vi "DebugProg.vi"() -> ()   [LabVIEW 2010]
uses:
  Instance           5 17Saved   DebugProg .vi
panel:
  out "Array":u8[](array[numeric])
  out "Result Input FOR VOC":u8[](array[numeric])
  out "ALG MSG  PARAM 2":enum16{"void", "byte", "int", "float"}(ring)
  out "Output varables names":string[](array[string])
  out "Output varables type":string[](array[string])
  out "AY Input varables names":string[](array[string])
  out "AY Input varables type":string[](array[string])
  out "Output ALG Msg Last Iter":string[][](table)=[["CODE", "PARAM"]]
  out "Output VOC Msg Last Iter":string[][](table)=[["CODE", "PARAM"]]
  out "Curr step ALG msg counter":i32
  out "Curr step VOC MSG counter":i32
  in  "Mode":bool
  in  "stop 2":bool
  in  "run":bool
  in  "Tab Control":T1(tab)=enum."Output ALG Info"
  out "ALG MSG queue":i32(slide) scale=0.0..5.0
  in  "send ALG msg":bool
  in  "ALG MSG  PARAM":string
  in  "ALG MSG  CODE":string(combo)="1"
  out "VOC MSG queue":i32(slide) scale=0.0..5.0
  in  "send voc msg 2":bool
  in  "VOC MSG  PARAM":string
  in  "VOC MSG  CODE":string(combo)
  in  "ALG MSG  TYPE":enum16{"void", "byte", "int", "float"}(ring)
  in  "VOC MSG  TYPE":enum16{"void", "byte", "int", "float"}(ring)
  out "AY OUTPUT Variables":string[][](table)
  in  "AY INPUT Variables":string[][](table)
  in  "New value\n(ALG ports)":u8
  in  "Controlable\n(ALG ports)":bool
  in  "Set new value\n(ALG ports)":bool
  in  "ALG Input Ports":i32(listbox)
  out "VOC OUTPUT Variables":string[][](table)
  in  "New value (VOC ports)":u8
  in  "Controlable (VOC ports)":bool
  in  "Set new value (VOC ports)":bool
  in  "VOC Input Ports":i32(listbox)
  in  "VOC INPUT Variables":string[][](table)
  in  "ALG Last Interation MSG":i32(listbox)
  out "Alg States":string[][](table)=[["Инициализация", "Начало", "0"], ["ОстановВсехПроцессовИстартПроцИнициализация", "Начало", "0"], ["КонтрольДостоверностиДавленияВбакеКомпрессора", "Начало", "0"], ["КонтрольДостоверностиДавленияВпатрубке", "Начало", "0"], ["КонтрольДостоверностиТемпературыВрубашкеОхлаждения", "Начало", "0"], ["КонтрольДостоверностиТемпературыВбакеОхлаждения", "Начало", "0"], ["КонтрольДостоверностиДавленияВтрубеСидеростата", "Начало", "0"], ["КонтрольДостоверностиСостоянияПитанияШКАФА_ВС", "Начало", "0"], ["КонтрольДостоверностиОткрЗатВакуумного", "Начало", "0"], ["КонтрольДостоверностиЗакрЗатВакуумного", "Начало", "0"], ["КонтрольДостоверностиСостоянияСапуна", "Начало", "0"], ["КонтрольДостоверностиСостоянияУстройстваПлавПуска", "Начало", "0"], ["КонтрольДостоверностиСостПитанияУППВакНасоса", "Начало", "0"], ["КонтрольДостоверностиСостоянияПитанияВентилятора", "Начало", "0"], ["КонтрольДостоверностиСостоянияПитанияРегТемпературы", "Начало", "0"], ["КонтрольДостоверностиСостоянияПитанияРегУровня", "Начало", "0"], ["КонтрольДостоверностиУровняВодыМинимум", "Начало", "0"], ["КонтрольДостоверностиУровняВодыМаксимум", "Начало", "0"], ["КонтрольДостоверностиСостоянияПитанияНасОхлаждения", "Начало", "0"], ["ЧтениеДавленияВбакеКомпрессора", "Начало", "0"], ["ОтлючитьВакуумированиеВручную", "ПереходВручноеОтключение", "0"], ["ЧтениеДавленияВпатрубке", "Начало", "0"], ["ЧтениеТемпературыВрубашкеОхлаждения", "Начало", "0"], ["ЧтениеТемпературыВбакеОхлаждения", "Начало", "0"], ["ЧтениеДавленияВтрубеСидеростата", "Начало", "0"], ["ПроверкаСвязиС_РегуляторомУровня", "Начало", "0"], ["ПроверкаСвязиС_РегуляторомТемпературы", "Начало", "0"], ["ПроверкаСвязиС_Вентилятором", "Начало", "0"], ["ПроверкаСвязиС_НасососомОхлажденияДвигателя", "Начало", "0"], ["ПроверкаСвязиС_КонцевикомОткрытияЗатвораВакуумного", "Начало", "0"], ["ПроверкаСвязиС_КонцевикомЗакрытияЗатвораВакуумного", "Начало", "0"], ["ПроверкаСвязиС_КонцевикомСапуна", "Начало", "0"], ["ПроверкаСвязиС_ПитаниемПлавногоПуска", "Начало", "0"], ["ПроверкаСвязиС_ПлавнымПуском", "Начало", "0"], ["РЕГУЛЯТОР_ТРАФИКА", "Начало", "0"], ["ЧтениеКольцевогоБуфера", "Начало", "0"], ["ОбработкаКомандИзмененияНП_от_ГУИ", "Анализ", "0"], ["ОбработкаКомандУправления_от_ГУИ", "Анализ", "0"], ["КонтрольИзменения_ФП_P_ВбакеКомпрессора", "Начало", "0"], ["КонтрольИзменения_ФП_P_Впатрубке", "Начало", "0"], ["КонтрольИзменения_ФП_T_Врубашке", "Начало", "0"], ["КонтрольИзменения_ФП_T_Вбаке", "Начало", "0"], ["КонтрольИзменения_ФП_P_ВтрубеСидер", "Начало", "0"], ["КонтрольВеличиныОткачкиВауумнойТрубыСидеростата", "Начало", "0"], ["КонтрольГотовностиВакуума_в_Вакуумной_Трубе", "Начало", "0"], ["КонтрольУровняВодыБакаОхлаждения", "Начало", "0"], ["КонтрольТемпературыВодыБакаОхлаждения", "Начало", "0"], ["КонтрольТемпературыРубашкиОхлаждения", "Начало", "0"], ["КонтрольДавленияВбакеКомпрессора", "Начало", "0"], ["КонтрольАварийногоДавленияВбакеКомпрессора", "Начало", "0"], ["КонтрольАварийнойТемпературыВрубашкеОхлаждения", "Начало", "0"], ["КонтрольАварийнойТемпературыВбакеОхлаждения", "Начало", "0"], ["КонтрольСостоянияПитанияШКАФА_ВС", "Начало", "0"], ["КонтрольСостоянияОборудования", "КонтрольОборудования", "0"], ["ВКЛ_ПИТ_ВЕНТИЛЯТОР", "Начало", "0"], ["ВЫК_ПИТ_ВЕНТИЛЯТОР", "Начало", "0"], ["КонтрольСостоянияПитанияВентилятора", "Начало", "0"], ["КонтрольСпонтанногоВыключенияВентилятора", "Контроль", "0"], ["КонтрольСпонтанногоВключенияВентилятора", "Контроль", "0"], ["КонтрольСостоянияЗатвораВакуумного", "Начало", "0"], ["ОТКР_ЗАТВОР_ВАК", "Начало", "0"], ["ЗАКР_ЗАТВОР_ВАК", "Начало", "0"], ["КонтрольСпонтанногоЗакрытияЗатвораВакуумного", "КонтрольЗакрытия", "0"], ["КонтрольСпонтанногоОткрытияЗатвораВакуумного", "Контроль", "0"], ["ОТКР_САПУН", "Начало", "0"], ["ЗАКР_САПУН", "Начало", "0"], ["КонтрольСостоянияПитанияСапуна", "Начало", "0"], ["КонтрольСпонтанногоЗакрытияСапуна", "КонтрольЗакрытия", "0"], ["КонтрольСпонтанногоОткрытияСапуна", "Контроль", "0"], ["ВКЛ_ПИТ_УПП_ВАК_НАСОСА", "Начало", "0"], ["ВЫК_ПИТ_УПП_ВАК_НАСОСА", "Начало", "0"], ["КонтрольСостоянияПитанияУППВакНасоса", "Начало", "0"], ["КонтрольСпонтанногоВыключенияУППВакНасоса", "Контроль", "0"], ["КонтрольСпонтанногоВключенияУППВакНасоса", "Контроль", "0"], ["ВКЛ_ПИТ_РЕГ_Т", "Начало", "0"], ["ВЫК_ПИТ_РЕГ_Т", "Начало", "0"], ["КонтрольСостоянияПитанияРЕГ_Т", "Начало", "0"], ["КонтрольСпонтанногоВыключенияРЕГ_Т", "Контроль", "0"], ["КонтрольСпонтанногоВключенияРЕГ_Т", "Контроль", "0"], ["ВКЛ_ПИТ_РЕГ_УР", "Начало", "0"], ["ВЫК_ПИТ_РЕГ_УР", "Начало", "0"], ["КонтрольСостоянияПитанияРЕГ_УР", "Начало", "0"], ["КонтрольСпонтанногоВыключенияРЕГ_УР", "Контроль", "0"], ["КонтрольСпонтанногоВключенияРЕГ_УР", "Контроль", "0"], ["ВКЛ_ПИТ_НАС_ОХЛ", "Начало", "0"], ["ВЫК_ПИТ_НАС_ОХЛ", "Начало", "0"], ["КонтрольСостоянияПитанияНАС_ОХЛ", "Начало", "0"], ["КонтрольСпонтанногоВыключенияНасосаОхлаждения", "Контроль", "0"], ["КонтрольСпонтанногоВключенияНасосаОхлаждения", "Контроль", "0"], ["ВКЛ_УСТР_ПЛАВ_ПУСКА", "Начало", "0"], ["ВЫК_УСТР_ПЛАВ_ПУСКА", "Начало", "0"], ["КонтрольСостоянияПитанияПЛАВ_ПУСКА", "Начало", "0"], ["КонтрольСпонтанногоВыключенияПлавнПуска", "Контроль", "0"], ["КонтрольСпонтанногоВключенияПлавнПуска", "Контроль", "0"], ["ВКЛ_ВАКУУМИРОВАНИЕ_ТРУБЫ", "Начало", "0"], ["ВЫК_ВАКУУМИРОВАНИЕ_ТРУБЫ", "Начало", "0"], ["ВКЛ_ВАКУУМНЫЙ_НАСОС", "Начало", "0"], ["ВЫК_ВАКУУМНЫЙ_НАСОС", "Начало", "0"]]
  out "Output Alg Msg LOG":string[][](table)=[["CODE", "PARAM"]]
  in  "VOC Last Interation MSG":i32(listbox)
  out "Output VOC Msg LOG":string[][](table)=[["CODE", "PARAM"]]
  out "VOC States":string[][](table)
  in  "Save as new test":bool
  in  "Save changes in current test":bool
  in  "TEST":string="script_port: 8 /*index*/, 0 /* СЦЕНАРИЙ_ЛОГ_ВХОД_ПИТ_ВЕНТИЛЯТОРА*/ \r\nscript_port: 9 /*index*/, 0 /* СЦЕНАРИЙ_ЛОГ_ВХОД_ПИТ_РЕГ_Т*/ \r\nscript_port: 10 /*index*/, 0 /* СЦЕНАРИЙ_ЛОГ_ВХОД_НАС_ОХЛ*/ \r\nscript_port: 11 /*index*/, 0 /* СЦЕНАРИЙ_ЛОГ_ВХОД_ВАК_НАСОСА*/ \r\nscript_port: 12 /*index*/, 0 /* СЦЕНАРИЙ_ЛОГ_ВХОД_ЗАТВОР_ВАК*/ \r\nscript_port: 13 /*index*/, 0 /* СЦЕНАРИЙ_ЛОГ_ВХОД_САПУН*/ \r\nscript_port: 14 /*index*/, 0 /* СЦЕНАРИЙ_ЛОГ_ВХОД_УСТР_ПЛАВ_ПУСКА*/ \r\nscript_port: 15 /*index*/, 0 /* СЦЕНАРИЙ_ЛОГ_ВХОД_РЕГ_УР*/ \r\nscript_port: 16 /*index*/, 0 /* СЦЕНАРИЙ_ЛОГ_ВХОД_КОМПРЕССОР*/ \r\n\n\n\n\n\n\n\n"
  in  "Tests List":i32(listbox)
  in  "stop":bool
  # "STEP MODE"
  # "CONTINUOUS MODE"
  # "ALG MSG Generation"
  # "VOC MSG Generation"
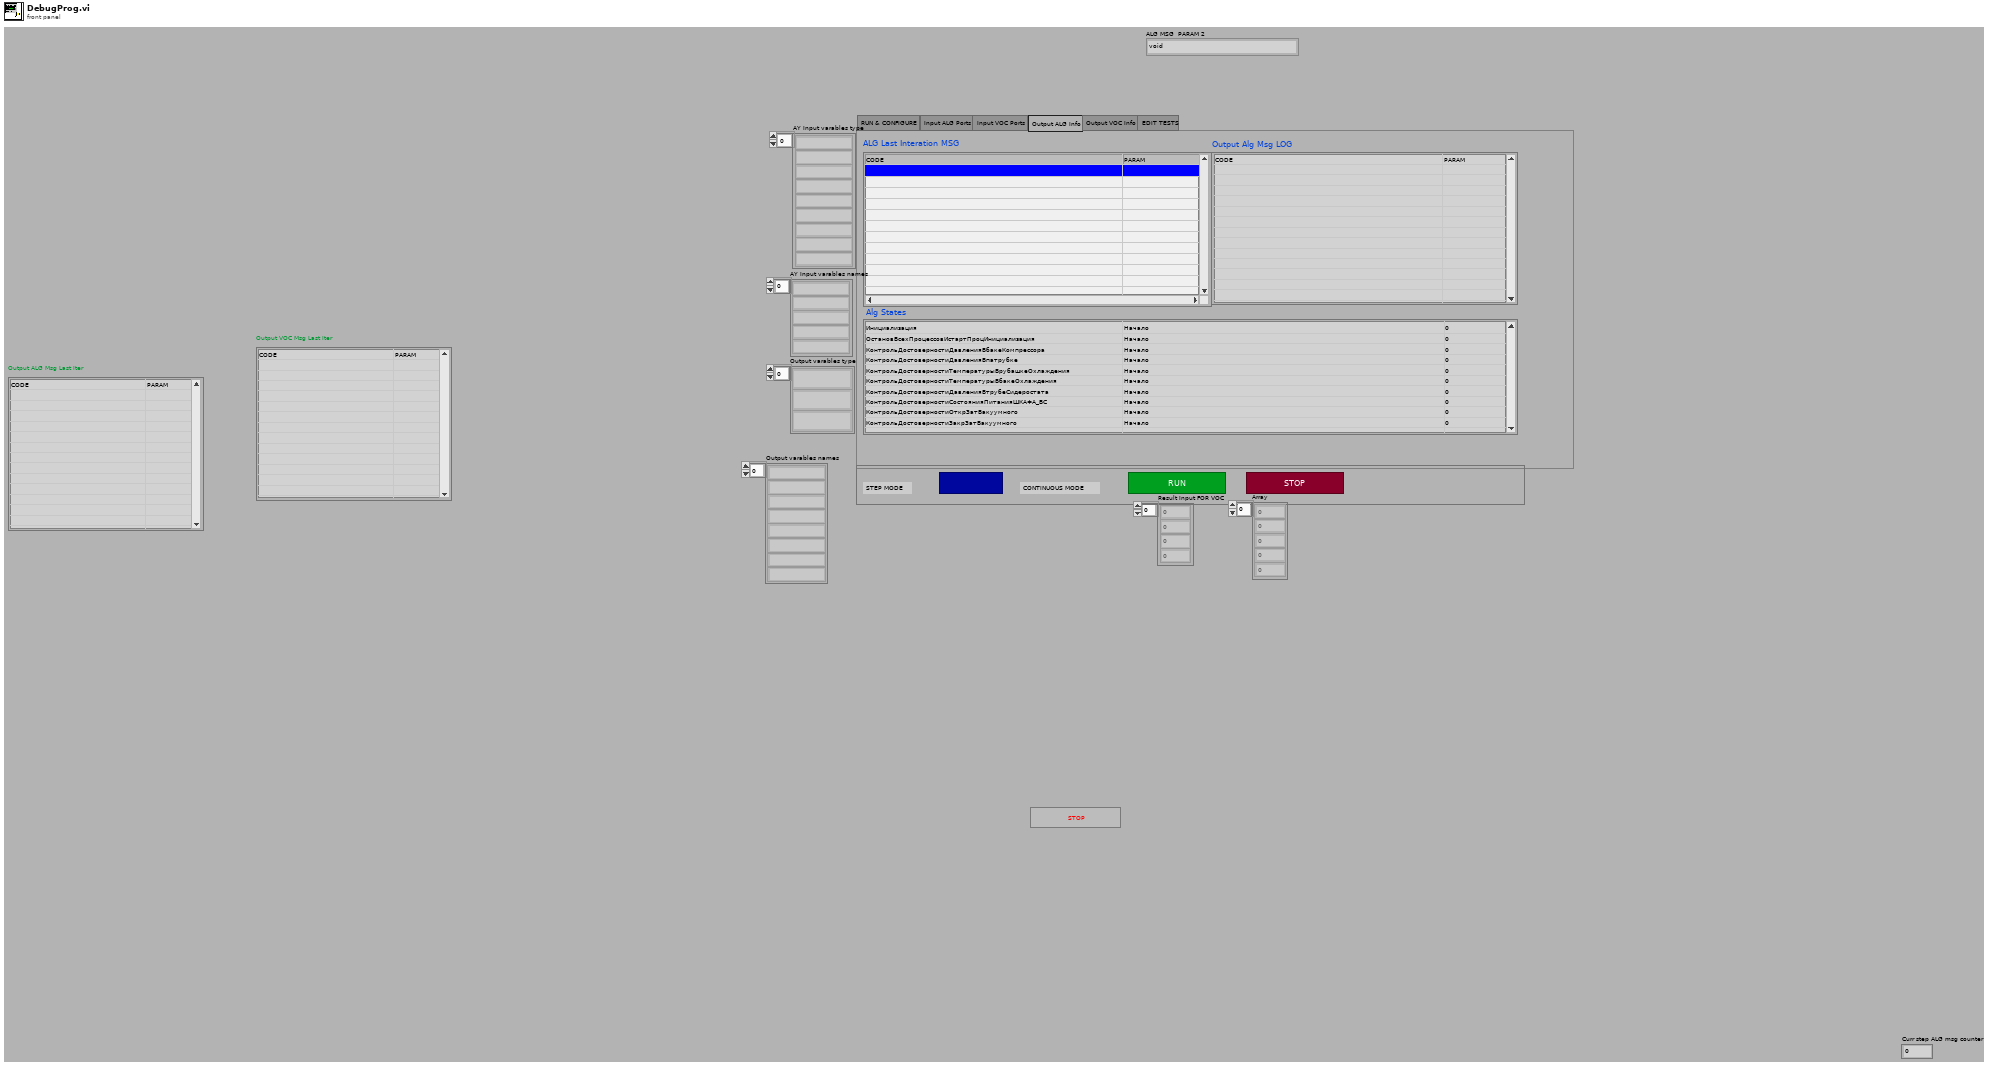
[diagram p1: front panel]
types:
  T1 = enum32{"RUN & CONFIGURE", "Input ALG Ports", "Input VOC Ports ", "Output ALG Info", "Output VOC Info", "EDIT TESTS"}
  T2 = enum8{"Enabled", "Disabled", "Disabled and Grayed Out"}
  T3 = enum16{"open", "open or create", "create or replace", "create", "open (read only)"}
  T4 = cluster{"code":i32, "param":i32, "Enum":enum16{"void", "byte", "int", "float"}}
  T5 = cluster{"trimmed string":string, "trimmed string":string}[]
  T6 = cluster{"code":i32, "param":i32, "Enum":enum16{"void", "byte", "int", "float"}}[]
  T7 = cluster{i32, "Casted Parameter":i32, "ALG MSG  TYPE":enum16{"void", "byte", "int", "float"}}
  T8 = cluster{i32, "Casted Parameter":i32, "VOC MSG  TYPE":enum16{"void", "byte", "int", "float"}}
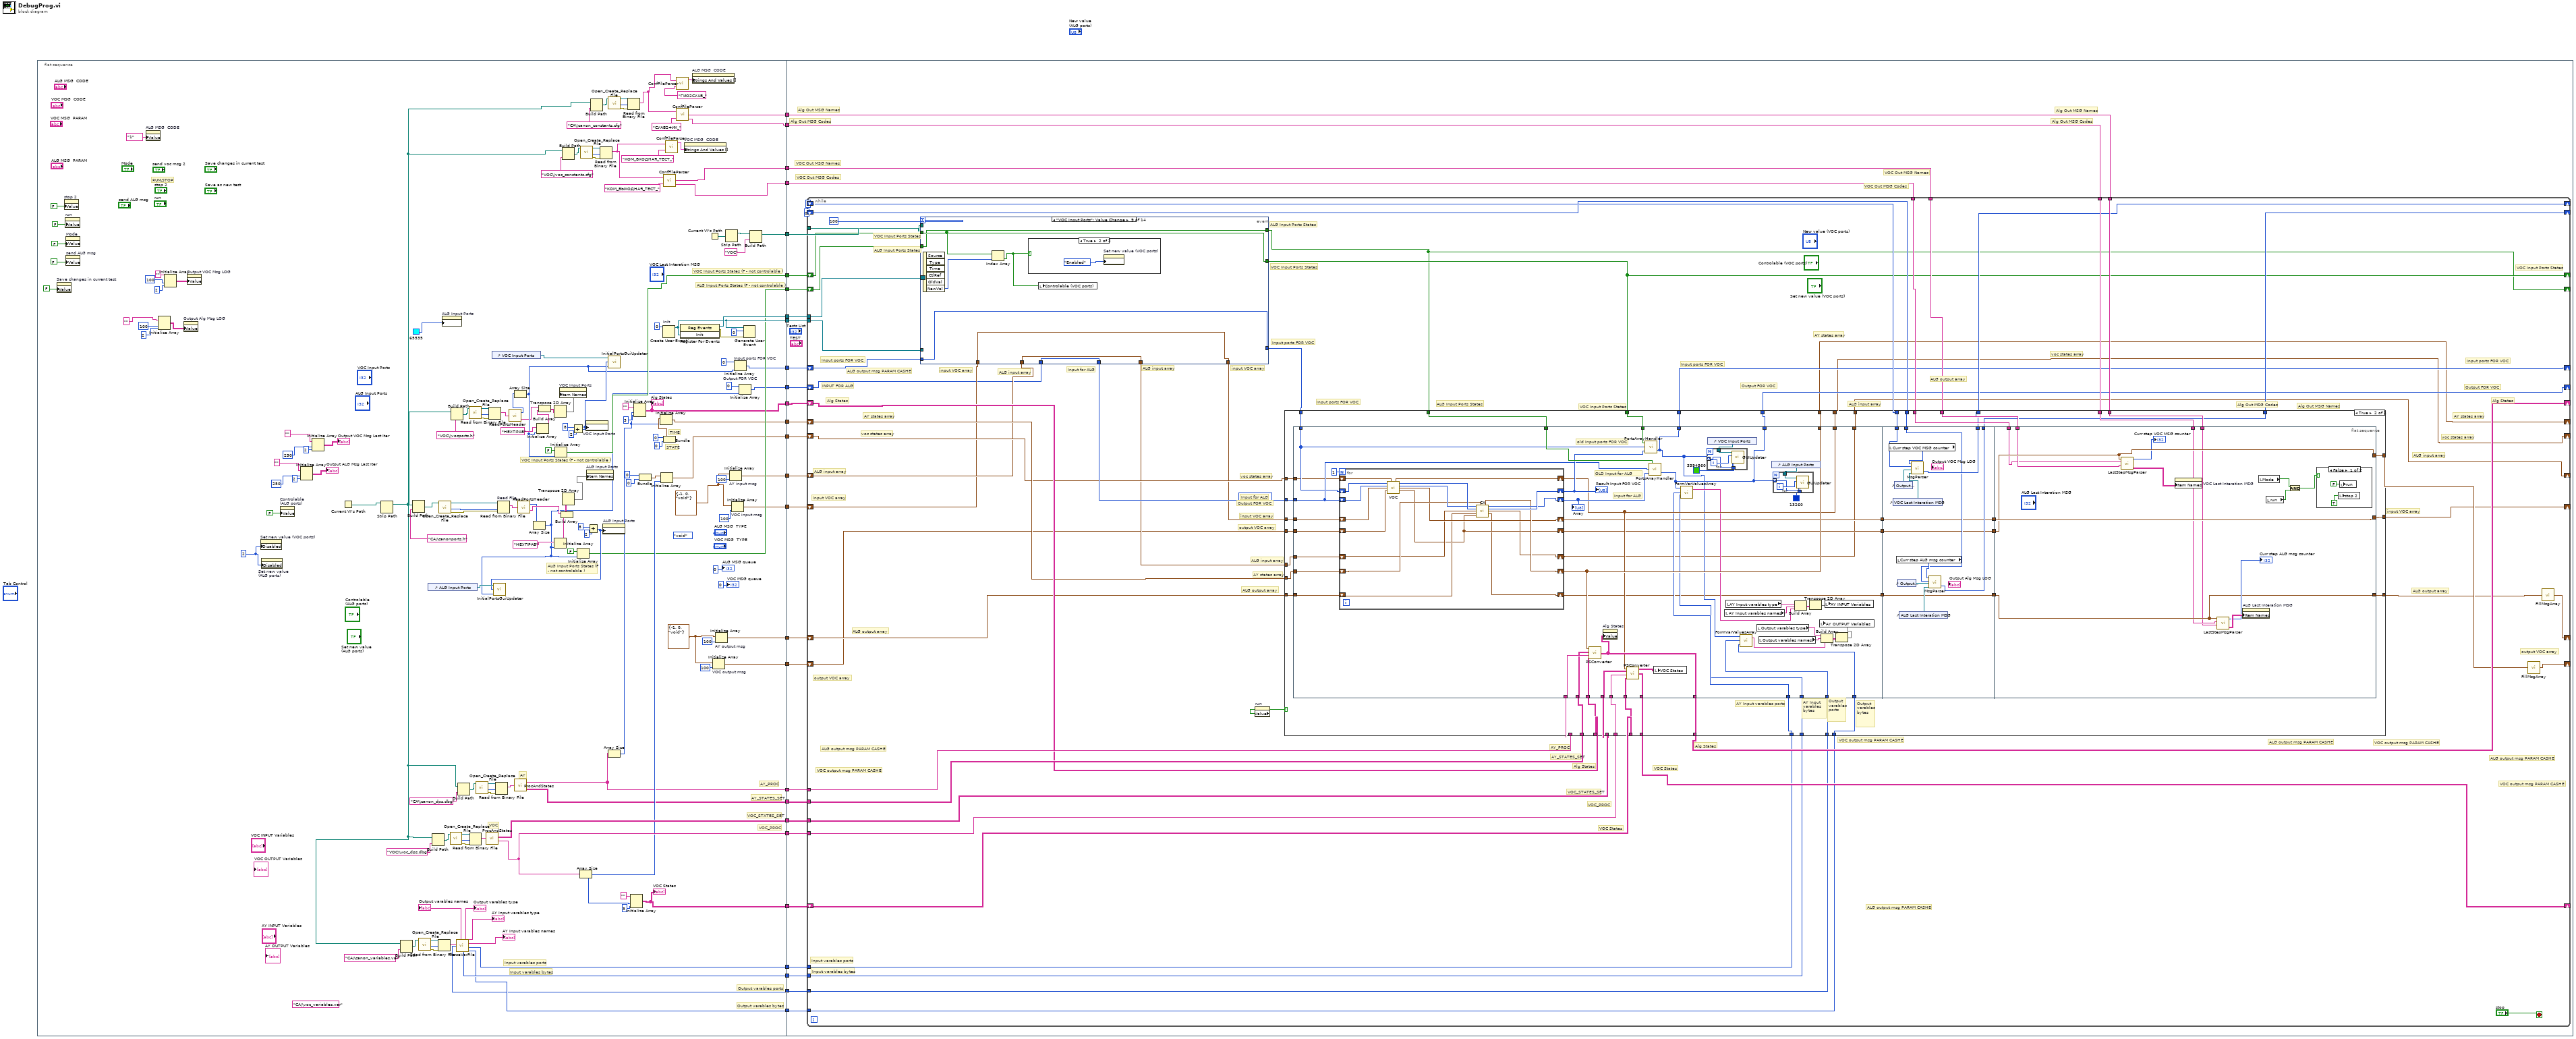
[diagram p0: block diagram]
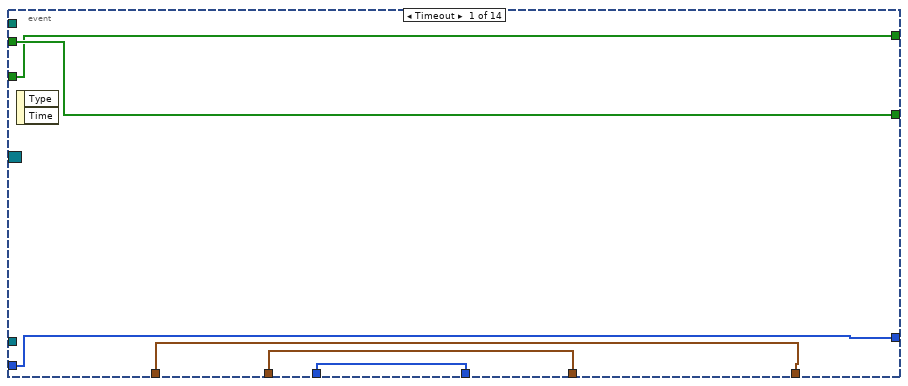
[diagram p2: hidden frame]
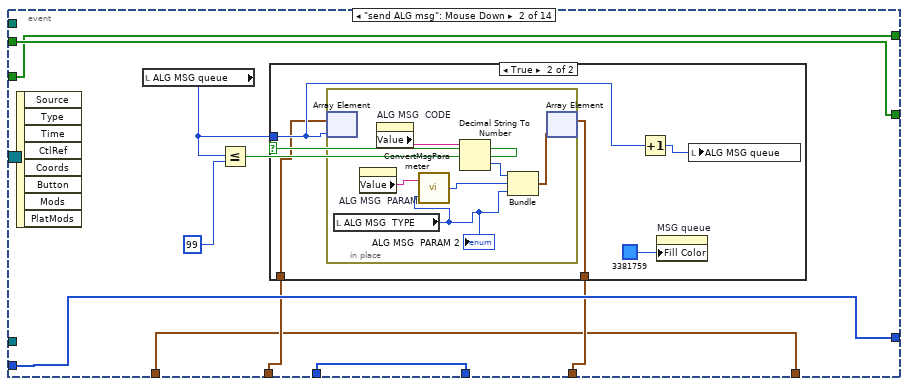
[diagram p3: hidden frame]
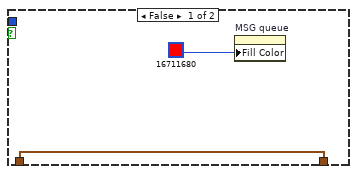
[diagram p4: hidden frame]
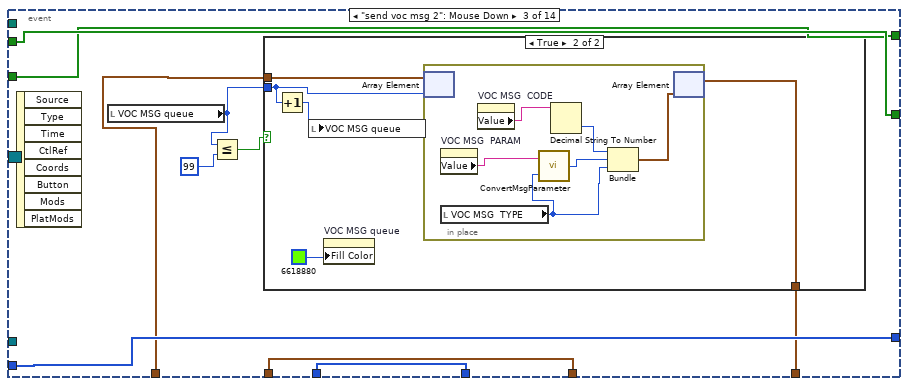
[diagram p5: hidden frame]
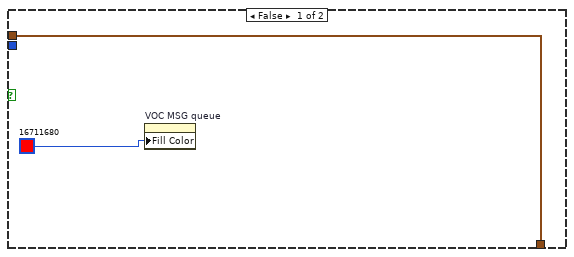
[diagram p6: hidden frame]
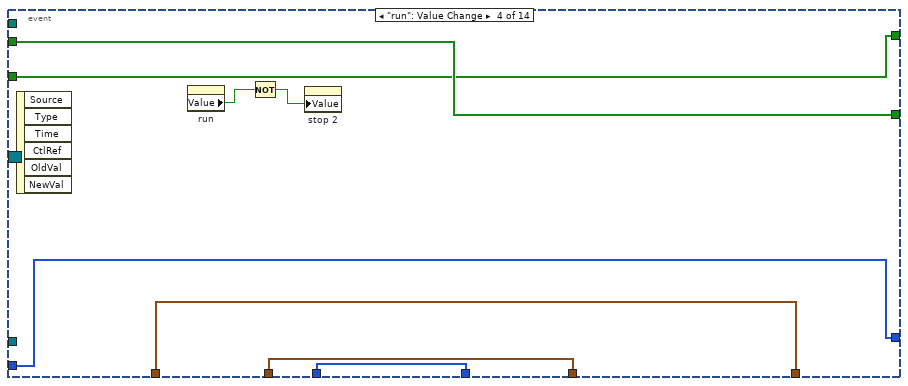
[diagram p7: hidden frame]
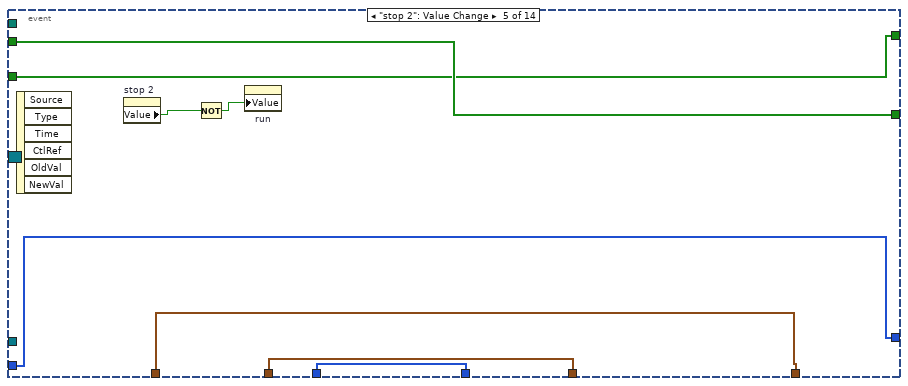
[diagram p8: hidden frame]
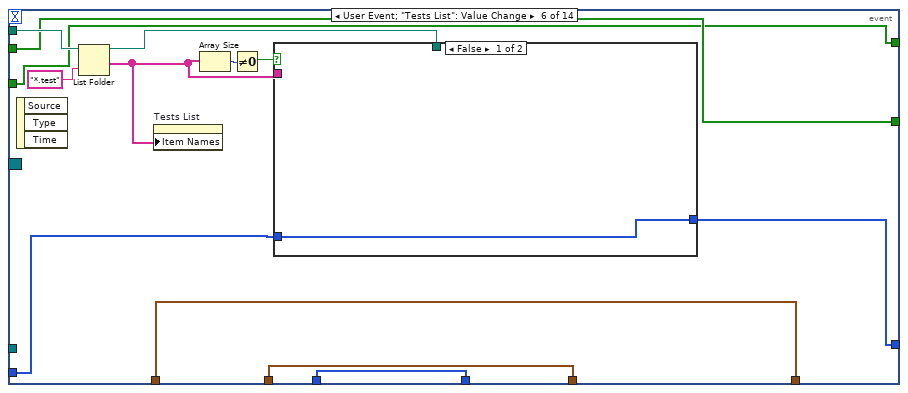
[diagram p9: hidden frame]
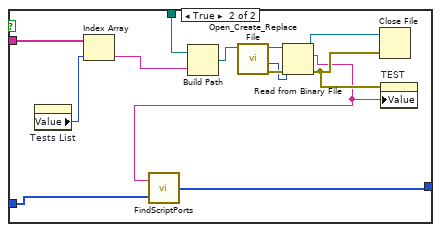
[diagram p10: hidden frame]
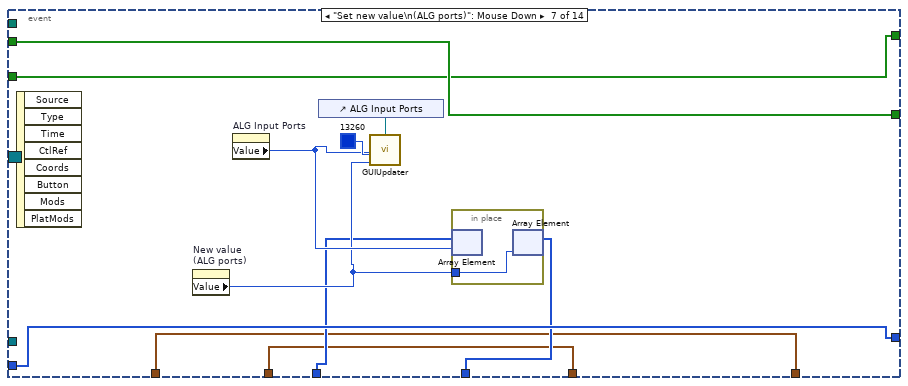
[diagram p11: hidden frame]
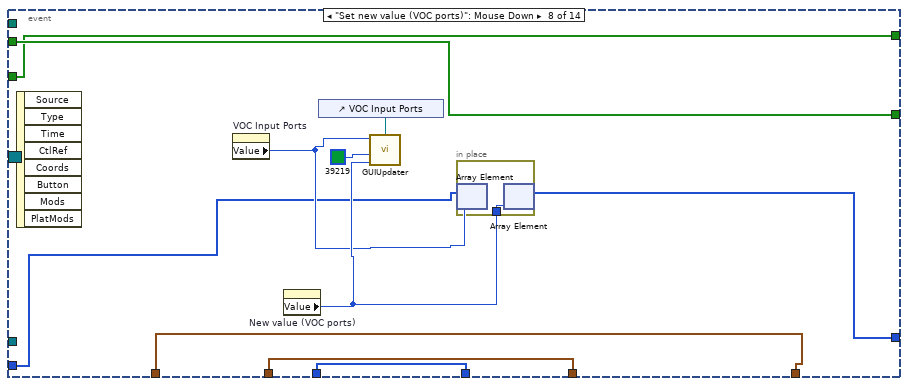
[diagram p12: hidden frame]
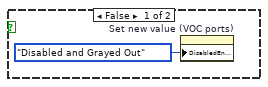
[diagram p13: hidden frame]
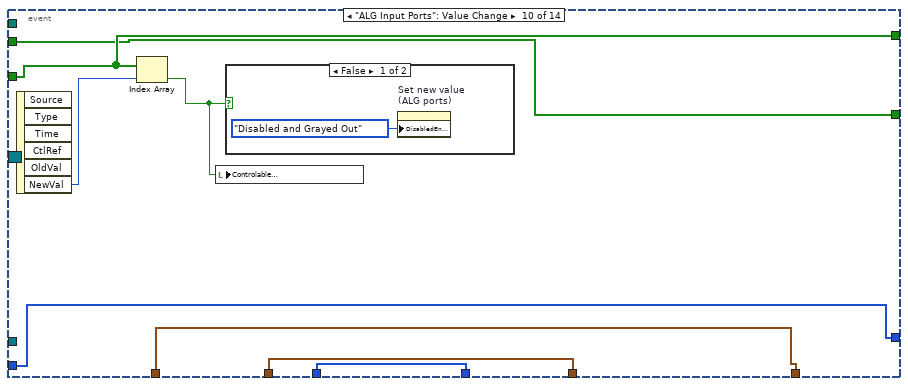
[diagram p14: hidden frame]
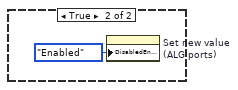
[diagram p15: hidden frame]
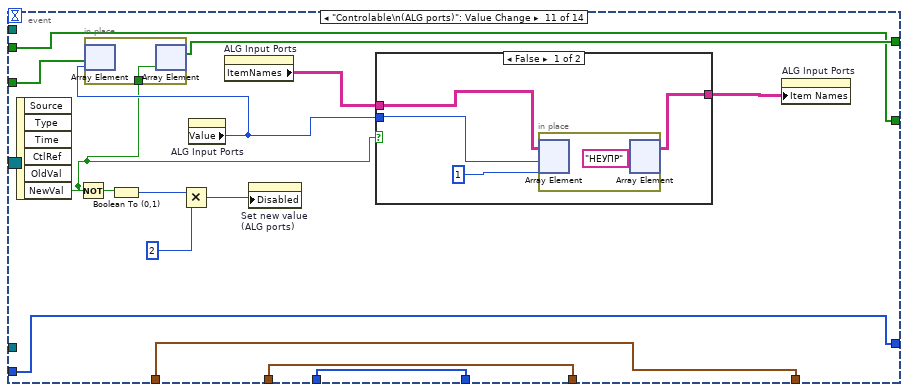
[diagram p16: hidden frame]
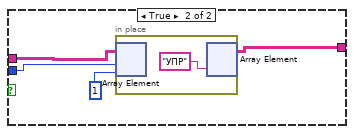
[diagram p17: hidden frame]
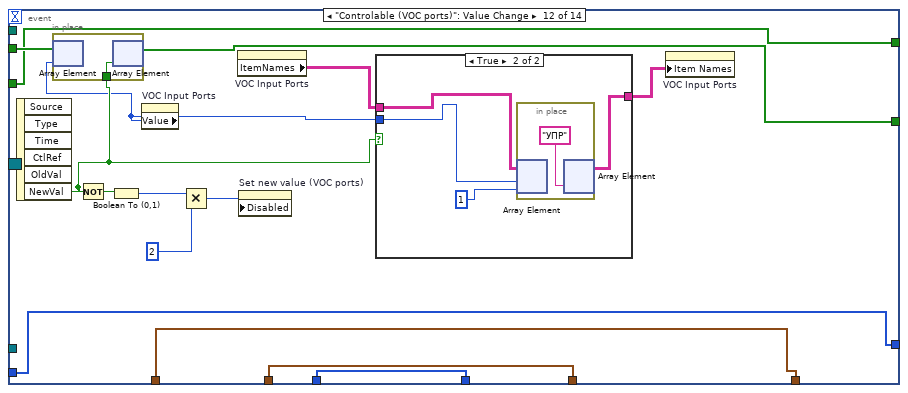
[diagram p18: hidden frame]
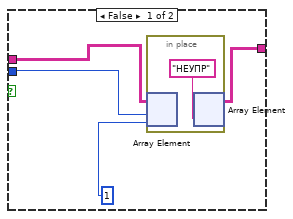
[diagram p19: hidden frame]
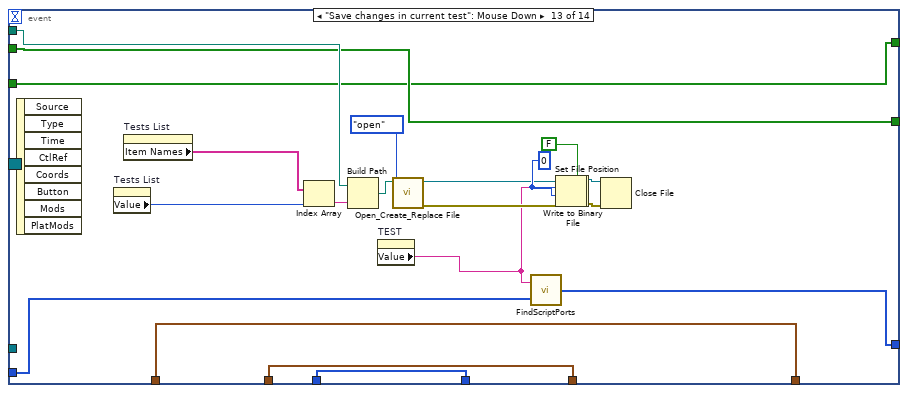
[diagram p20: hidden frame]
diagram:
  n1 = flat-sequence {
    tunnel: [w137] -> w27
    tunnel: [w131] -> w26
    tunnel: [w133] -> w25
    tunnel: [w129] -> w24
    tunnel: [w128] -> w23
    tunnel: [w127] -> w22
    tunnel: [w126] -> w21
    tunnel: [w74] -> w20
    tunnel: [w73] -> w19
    tunnel: [w109] -> w18
    tunnel: [w112] -> w17
    tunnel: [w70] -> w16
    tunnel: [w68] -> w15
    tunnel: [w65] -> w14
    tunnel: [w64] -> w13
    tunnel: [w63] -> w12
    tunnel: [w62] -> w11
    tunnel: [w61] -> w10
    tunnel: [w60] -> w9
    tunnel: [w59] -> w8
    tunnel: [w58] -> w7
    tunnel: [w57] -> w6
    tunnel: [w56] -> w5
    tunnel: [w40] -> w4
    tunnel: [w49] -> w3
    tunnel: [w28] -> w2
    tunnel: [w48] -> w1
    tunnel: w27 -> [w214]
    tunnel: w26 -> [w213]
    tunnel: w25 -> [w212]
    tunnel: w24 -> [w209]
    tunnel: w23 -> [w208]
    tunnel: w22 -> [w211]
    tunnel: w21 -> [w210]
    tunnel: w20 -> [w206]
    tunnel: w19 -> [w205]
    tunnel: w18 -> [w204]
    tunnel: w17 -> [w203]
    tunnel: w16 -> [w201]
    tunnel: w15 -> [w200]
    tunnel: w14 -> [w199]
    tunnel: w13 -> [w198]
    tunnel: w12 -> [w197]
    tunnel: w11 -> [w196]
    tunnel: w10 -> [w195]
    tunnel: w9 -> [w189]
    tunnel: w8 -> [w188]
    tunnel: w7 -> [w187]
    tunnel: w6 -> [w186]
    tunnel: w5 -> [w194]
    tunnel: w4 -> [w193]
    tunnel: w3 -> [w192]
    tunnel: w2 -> [w191]
    tunnel: w1 -> [w190]
    frame #0 {
      (unwired) "CA\\voc_variables.var" ("name or relative path")
      (unwired) enum16{"void", "byte", "int", "float"}."void" ("Enum")
      w41 = T4 {"code"=-1, "param"=0, "Enum"=enum."void"} ("Cluster")
      w42 = T4 {"code"=-1, "param"=0, "Enum"=enum."void"} ("Cluster")
      w76 = u8 2 ("Disabled")
      w136 = 0  # Init
      # "Output varables bytes"
      # "Output varables ports"
      # "Input varables bytes"
      # "Input varables ports"
      # "VOC Input Ports States (F - not controlable )"
      # "ALG Input Ports States (F - not controlable )"
      # "VOC Input Ports States (F - not controlable )"
      # "ALG Input Ports States (F - not controlable )"
      # "AY"
      # "VOC"
      # "VOC_STATES_SET"
      # "VOC_PROC"
      # "AY_STATES_SET"
      # "AY_PROC"
      # "STATE"
      # "TIME"
      # "RUN\\STOP"
      n2 = property on="Save changes in current test" class="Bool (strict)"("Value"=FALSE ("Save changes in current test")) -> ()  [unwired: 2 in, 2 out]
      n3 = property on="stop 2" class="Bool (strict)"("Value"=FALSE ("send msg 3")) -> ()  [unwired: 2 in, 2 out]
      n4 = property on="run" class="Bool (strict)"("Value"=FALSE ("send msg 2")) -> ()  [unwired: 2 in, 2 out]
      n5 = property on="Mode" class="Bool (strict)"("Value"=FALSE ("Mode")) -> ()  [unwired: 2 in, 2 out]
      n6 = property on="send ALG msg" class="Bool (strict)"("Value"=FALSE ("send msg")) -> ()  [unwired: 2 in, 2 out]
      n7 = property on="ALG MSG  CODE" class="CmbBox"("Value"="1" ("CODE")) -> ()  [unwired: 2 in, 2 out]
      n8 = Initialize Array("" ("element"), 100 ("dimension size"), 2 ("dimension size")) -> (w117:string[][])
      n9 = Initialize Array("" ("element"), 100 ("dimension size"), 2 ("dimension size")) -> (w118:string[][])
      n10 = property on="Output Alg Msg LOG" class="Tbl (strict)"("Value"=w117) -> ()  [unwired: 2 in, 2 out]
      n11 = property on="Output VOC Msg LOG" class="Tbl (strict)"("Value"=w118) -> ()  [unwired: 2 in, 2 out]
      n12 = property on="Set new value (VOC ports)" class="Bool (strict)"("Disabled"=w76) -> ()  [unwired: 2 in, 2 out]
      n13 = property on="Set new value\n(ALG ports)" class="Bool (strict)"("Disabled"=w76) -> ()  [unwired: 2 in, 2 out]
      n14 = property on="Controlable\n(ALG ports)" class="Bool (strict)"("Value"=FALSE ("Controlable")) -> ()  [unwired: 2 in, 2 out]
      n15 = Initialize Array("" ("Value"), 250 ("dimension size"), 2 ("dimension size")) -> (→"Output ALG Msg Last Iter":string[][])
      n16 = Initialize Array("" ("Value"), 250 ("dimension size"), 2 ("dimension size")) -> (→"Output VOC Msg Last Iter":string[][])
      n17 = Current VI's Path() -> (path=w125:path)
      n18 = Strip Path(path=w125) -> (stripped path=w29:path)  [unwired: 1 out]
      n19 = Build Path(base path=w29, name or relative path="CA\\canon_variables.var") -> (appended path=w53:path)
      n20 = Build Path(base path=w29, name or relative path="CA\\canonports.h") -> (appended path=w99:path)
      n21 = call <vilib>:"Open_Create_Replace File.vi"("file path"=w53) -> ("error out"=w55:errorcluster, "file size (bytes)"=w54:i32, "refnum"=w43:refnum<file>)  [unwired: 7 in, 1 out]
      n22 = control-ref of="ALG Input Ports"() -> (w80:refnum<vi>)
      n23 = Build Path(base path=w29, name or relative path="VOC\\voc_dps.dbg") -> (appended path=w158:path)
      n24 = Read from Binary File(8:w55, 10:w54, 11:w43) -> (2:w52:string)  [unwired: 3 in, 3 out]
      n25 = call <vilib>:"Open_Create_Replace File.vi"("file path"=w99) -> ("error out"=w98:errorcluster, "file size (bytes)"=w97:i32, "refnum"=w96:refnum<file>)  [unwired: 7 in, 1 out]
      n26 = property on="ALG Input Ports" class="MCListbox (strict)"("Selection Color"=u32 65535) -> ()  [unwired: 2 in, 2 out]
      n27 = call <vilib>:"Open_Create_Replace File.vi"("file path"=w158) -> ("error out"=w157:errorcluster, "file size (bytes)"=w156:i32, "refnum"=w155:refnum<file>)  [unwired: 7 in, 1 out]
      n28 = Build Path(base path=w29, name or relative path="VOC\\vocports.h") -> (appended path=w89:path)
      n29 = call "ParseVarFile.vi"("data"=w52) -> ("Output varables bytes"=w48:i32[], "Output varables names"=→"Output varables names":string[], "Input varables ports"=w40:i32[], "Input varables names"=→"AY Input varables names":string[], "Output varables type"=→"Output varables type":string[], "Input varables type"=→"AY Input varables type":string[], "Input varables bytes"=w49:i32[], "Output varables ports"=w28:i32[])
      n30 = Build Path(base path=w29, name or relative path="CA\\canon_dps.dbg") -> (appended path=w150:path)
      n31 = call <vilib>:"Open_Create_Replace File.vi"("file path"=w89) -> ("error out"=w88:errorcluster, "file size (bytes)"=w87:i32, "refnum"=w86:refnum<file>)  [unwired: 7 in, 1 out]
      n32 = Read from Binary File(8:w157, 10:w156, 11:w155) -> (2:w130:string)  [unwired: 3 in, 3 out]
      n33 = call <vilib>:"Open_Create_Replace File.vi"("file path"=w150) -> ("error out"=w149:errorcluster, "file size (bytes)"=w148:i32, "refnum"=w147:refnum<file>)  [unwired: 7 in, 1 out]
      n34 = call "ProcAndStates.vi"("spreadsheet string"=w130) -> ("PROCESSES"=w109:string[], "STATES"=w112:string[][])
      n35 = Read from Binary File(8:w88, 10:w87, 11:w86) -> (2:w39:string)  [unwired: 3 in, 3 out]
      n36 = control-ref of="VOC Input Ports"() -> (w78:refnum<vi>)
      n37 = Read from Binary File(8:w149, 10:w148, 11:w147) -> (2:w160:string)  [unwired: 3 in, 3 out]
      n38 = Read from Binary File "Read File"(8:w98, 10:w97, 11:w96) -> (2:w34:string)  [unwired: 3 in, 3 out]
      n39 = call "ReadPortsHeader.vi"("data"=w39) -> ("Input Numbers"=w38:i32[], "Input Names"=w36:string[])
      n40 = Array Size(array=w38) -> (size(s)=w37:i32)
      n41 = call "ProcAndStates.vi"("spreadsheet string"=w160) -> ("PROCESSES"=w74:string[], "STATES"=w73:string[][])
      n42 = call "ReadPortsHeader.vi"("data"=w34) -> ("Input Numbers"=w31:i32[], "Input Names"=w33:string[])
      n43 = Array Size(array=w31) -> (size(s)=w30:i32)
      n44 = Initialize Array("НЕУПРАВ" ("name or relative path"), w37) -> (w83:string[])
      n45 = Build Array(w36, w83) -> (w82:string[][])
      n46 = Initialize Array("НЕУПРАВ" ("name or relative path"), w30) -> (w93:string[])
      n47 = Transpose 2D Array(2D array=w82) -> (transposed array=w69:string[][])
      n48 = Initialize Array(FALSE ("Controlable"), w37) -> (w68:bool[])
      n49 = property on="VOC Input Ports" class="MCListbox (strict)"("Item Names"=w69) -> ()  [unwired: 2 in, 2 out]
      n50 = Build Array(w33, w93) -> (w94:string[][])
      n51 = Build Path(base path=w29, name or relative path="VOC\\voc_constants.cfg") -> (appended path=w174:path)
      n52 = Transpose 2D Array(2D array=w94) -> (transposed array=w92:string[][])
      n53 = Add(x=8, y=2) -> (x+y=w77:i32)
      n54 = Initialize Array(FALSE ("Controlable"), w30) -> (w70:bool[])
      n55 = Array Size(array=w109) -> (size(s)=w108:i32)
      n56 = call <vilib>:"Open_Create_Replace File.vi"("file path"=w174) -> ("error out"=w173:errorcluster, "file size (bytes)"=w172:i32, "refnum"=w171:refnum<file>)  [unwired: 7 in, 1 out]
      n57 = property on="VOC Input Ports" class="MCListbox (strict)"("Number of Columns"=w77) -> ()  [unwired: 2 in, 2 out]
      n58 = property on="ALG Input Ports" class="MCListbox (strict)"("Item Names"=w92) -> ()  [unwired: 2 in, 2 out]
      n59 = Add(x=8, y=2) -> (x+y=w79:i32)
      n60 = call "InitialPortsGuiUpdater.vi"("Ports counter"=w30, "port max size"=w79, "MCListbox Refnum"=w80) -> ()
      n61 = Build Path(base path=w29, name or relative path="CA\\canon_constants.cfg") -> (appended path=w146:path)
      n62 = Read from Binary File(8:w173, 10:w172, 11:w171) -> (2:w176:string)  [unwired: 3 in, 3 out]
      n63 = property on="ALG Input Ports" class="MCListbox (strict)"("Number of Columns"=w79) -> ()  [unwired: 2 in, 2 out]
      n64 = Array Size(array=w74) -> (size(s)=w120:i32)
      n65 = call <vilib>:"Open_Create_Replace File.vi"("file path"=w146) -> ("error out"=w145:errorcluster, "file size (bytes)"=w144:i32, "refnum"=w143:refnum<file>)  [unwired: 7 in, 1 out]
      n66 = call "InitialPortsGuiUpdater.vi"("Ports counter"=w37, "port max size"=w77, "MCListbox Refnum"=w78) -> ()
      n67 = Read from Binary File(8:w145, 10:w144, 11:w143) -> (2:w167:string)  [unwired: 3 in, 3 out]
      n68 = Initialize Array("" ("Value"), w108, 3 ("dimension size")) -> (w56:string[][])
      "VOC States" <- w56
      n69 = Initialize Array("" ("Value"), w120, 3 ("dimension size")) -> (w63:string[][])
      "Alg States" <- w63
      n70 = Bundle(u32 0, u8 0) -> (w166:cluster{u32, u8})  [unwired: 1 in]
      n71 = Initialize Array(w166, w108) -> (w61:cluster{u32, u8}[])
      n72 = Create User Event(user event datatype=w136) -> (user event=w131:refnum<user-event>)  [unwired: 1 in, 1 out]
      n73 = call "ConfFileParser.vi"("TEXT"=w176, "search string"="КОМ_ВЫХОДНАЯ_ТЕСТ_") -> ("Names"=w127:string[], "Codes"=w126:string[])  [unwired: 1 out]
      n74 = Bundle(u32 0, u8 0) -> (w163:cluster{u32, u8})  [unwired: 1 in]
      n75 = Initialize Array(w163, w120) -> (w62:cluster{u32, u8}[])
      n76 = call "ConfFileParser.vi"("TEXT"=w176, "search string"="КОМ_ВХОДНАЯ_ТЕСТ_") -> ("Cluster Array"=w169:T5)  [unwired: 2 out]
      n77 = call "ConfFileParser.vi"("TEXT"=w167, "search string"="ГИО2СУАБ_") -> ("Cluster Array"=w152:T5)  [unwired: 2 out]
      n78 = call "ConfFileParser.vi"("TEXT"=w167, "search string"="СУАБ2ФИК_") -> ("Names"=w129:string[], "Codes"=w128:string[])  [unwired: 1 out]
      n79 = register-events(w131) -> (reference out=w133:refnum<event-registration>, error out=w135:errorcluster)  [unwired: 2 in]
      n80 = property on="VOC MSG  CODE" class="CmbBox"("Strings And Values []"=w169) -> ()  [unwired: 2 in, 2 out]
      n81 = property on="ALG MSG  CODE" class="CmbBox"("Strings And Values []"=w152) -> ()  [unwired: 2 in, 2 out]
      n82 = Current VI's Path() -> (path=w139:path)
      n83 = Initialize Array "VOC output msg"(w42, 100 ("dimension size")) -> (w57:T6)
      n84 = Initialize Array "AY output msg"(w42, 100 ("dimension size")) -> (w58:T6)
      n85 = Strip Path(path=w139) -> (stripped path=w138:path)  [unwired: 1 out]
      n86 = Initialize Array "AY input msg"(w41, 100 ("dimension size")) -> (w60:T6)
      n87 = Initialize Array "VOC input msg"(w41, 100 ("dimension size")) -> (w59:T6)
      n88 = Initialize Array "Input ports FOR VOC"(u8 0 ("element"), w37) -> (w65:u8[])
      n89 = Initialize Array "Output FOR VOC"(u8 0 ("element"), w30) -> (w64:u8[])
      n90 = Generate User Event(user event=w131, event data cluster=0, error in=w135) -> ()  [unwired: 2 out]
      n91 = Build Path(base path=w138, name or relative path="VOC") -> (appended path=w137:path)
      "VOC MSG queue" <- 0 ("VOC MSG queue")
      "ALG MSG queue" <- 0 ("ALG MSG queue")
    }
    frame #1 {
      # "VOC Out MSG Names"
      # "Alg Out MSG Codes"
      # "Alg Out MSG Names"
      # "VOC Out MSG Codes"
      # "VOC Out MSG Codes"
      # "VOC Out MSG Names"
      # "Alg Out MSG Codes"
      # "Alg Out MSG Names"
      n92 = while {
        tunnel: w214 -> [w262]
        tunnel: w213 -> [w264]
        tunnel: w212 -> [w265]
        tunnel: w211 -> [w261]
        tunnel: w210 -> [w260]
        tunnel: w209 -> [w258]
        tunnel: w208 -> [w259]
        shift-right: [w255] -> _
        shift-left: 0 -> [w256]
        tunnel: w204 -> [w252]
        tunnel: w206 -> [w254]
        tunnel: w205 -> [w253]
        tunnel: w203 -> [w249]
        shift-right: [w250] -> _
        shift-left: 0 -> [w251]
        shift-right: [w246] -> _
        shift-left: w200 -> [w247]
        shift-right: [w245] -> _
        shift-left: w201 -> [w248]
        shift-right: [w242] -> _
        shift-left: w199 -> [w244]
        shift-right: [w240] -> _
        shift-left: w198 -> [w215]
        shift-right: [w238] -> _
        shift-left: w197 -> [w239]
        shift-right: [w236] -> _
        shift-left: w196 -> [w237]
        shift-right: [w234] -> _
        shift-left: w195 -> [w235]
        shift-right: [w231] -> _
        shift-left: w194 -> [w230]
        tunnel: w193 -> [w227]
        tunnel: w192 -> [w226]
        tunnel: w191 -> [w225]
        tunnel: w190 -> [w224]
        shift-right: [w218] -> _
        shift-left: w189 -> [w223]
        shift-right: [w219] -> _
        shift-left: w188 -> [w222]
        shift-right: [w217] -> _
        shift-left: w187 -> [w221]
        shift-right: [w216] -> _
        shift-left: w186 -> [w220]
        stop <- "stop" stop-if-true
        # "Input varables bytes"
        # "Input varables ports"
        # "VOC Input Ports States"
        # "VOC Input Ports States"
        # "VOC Input Ports States"
        # "Input for ALG"
        # "ALG Input Ports States"
        # "ALG Input Ports States"
        # "ALG Input Ports States"
        # "VOC Input Ports States"
        # "Input for ALG"
        # "VOC output msg PARAM CASHE"
        # "VOC output msg PARAM CASHE"
        # "VOC output msg PARAM CASHE"
        # "VOC output msg PARAM CASHE"
        # "ALG output msg PARAM CASHE"
        # "ALG output msg PARAM CASHE"
        # "ALG output msg PARAM CASHE"
        # "ALG output msg PARAM CASHE"
        # "ALG output msg PARAM CASHE"
        # "voc states array"
        # "VOC States"
        # "Alg States"
        # "VOC States"
        # "Alg States"
        # "Alg States"
        # "Alg States"
        # "VOC_STATES_SET"
        # "VOC_PROC"
        # "AY_STATES_SET"
        # "AY_PROC"
        # "AY states array"
        # "ALG output array"
        # "ALG input array"
        # "output VOC array"
        # "ALG output array"
        # "input VOC array"
        # "ALG input array"
        # "voc states array"
        # "AY states array"
        # "Output FOR VOC"
        # "Input ports FOR VOC"
        # "Output FOR VOC"
        # "Input ports FOR VOC"
        # "Alg Out MSG Codes"
        # "Alg Out MSG Names"
        # "ALG output array"
        # "output VOC array"
        # "output VOC array"
        # "ALG output array"
        # "AY states array"
        # "voc states array"
        # "voc states array"
        # "AY states array"
        # "ALG input array"
        # "Output FOR VOC"
        # "INPUT FOR ALG"
        # "input VOC array"
        # "Input ports FOR VOC"
        # "input VOC array"
        # "ALG input array"
        # "input VOC array"
        # "input VOC array"
        # "Input ports FOR VOC"
        # "Input ports FOR VOC"
        # "ALG input array"
        # "ALG input array"
        n93 = event shown="[8] \"VOC Input Ports\": Value Change" {
          selector: w265 -> [_ _ _ _ _ _ _ _ _ _ _ _ _ _]
          dyn-events: _ -> [_ _ _ _ _ _ _ _ _ _ _ _ _ _]
          timeout: 100 -> [_ _ _ _ _ _ _ _ _ _ _ _ _ _]
          tunnel: w264 -> [_ _ _ _ _ _ _ _ _ _ _ _ _ _]
          tunnel: w262 -> [_ _ _ _ _ w343 _ _ _ _ _ _ w475 w488]
          tunnel: w248 -> [w271 w279 w302 w323 w331 w340 w367 w379 w390 w401 w411 w436 w463 w485]
          tunnel: [w271 w279 w302 w323 w331 w340 w367 w379 w390 w401 w412 w436 w463 w485] -> w245
          tunnel: w247 -> [w272 w280 w303 w324 w332 w341 w368 w380 w391 w400 w410 w440 w464 w486]
          tunnel: [w272 w280 w303 w324 w332 w341 w368 w380 w391 w400 w410 w437 w464 w486] -> w246
          tunnel: w244 -> [w270 w277 w300 w322 w330 w339 w366 w378 w389 w399 w409 w435 w462 w484]
          tunnel: [w270 w277 w300 w322 w330 w338 w366 w377 w389 w399 w409 w435 w461 w483] -> w243
          tunnel: w215 -> [w269 w276 w299 w321 w329 w337 w365 w376 w388 w398 w408 w434 w460 w482]
          tunnel: [w269 w276 w299 w321 w329 w337 w364 w376 w388 w398 w408 w434 w460 w482] -> w241
          tunnel: w223 -> [w268 w275 w298 w320 w328 w336 w363 w375 w387 w397 w407 w433 w459 w481]
          tunnel: [w268 w274 w298 w320 w328 w336 w363 w375 w387 w397 w407 w433 w459 w481] -> w233
          tunnel: w222 -> [w267 w273 w297 w319 w327 w335 w362 w374 w386 w396 w406 w432 w458 w480]
          tunnel: [w267 w273 w296 w319 w327 w335 w362 w374 w386 w396 w406 w432 w458 w480] -> w232
          event Timeout {
            n94 = event-data() -> ()  [unwired: 1 in, 2 out]
          }
          event "send ALG msg": Mouse Down {
            n95 = event-data() -> ()  [unwired: 1 in, 8 out]
            n96 = local read "ALG MSG queue"() -> (w278:i32)
            n97 = Less Or Equal?(x=w278, y=99) -> (x <= y?=w281:bool)
            n98 = case shown="True" w281 {
              tunnel: w278 -> [_ w288]
              tunnel: w275 -> [w283 w286]
              tunnel: [w283 w285] -> w274
              frame False {
                n99 = property on="MSG queue" class="Slide (strict)"("Fill Color"=u32 16711680) -> ()  [unwired: 2 in, 2 out]
              }
              frame True {
                n100 = in-place {
                  n101 = in-place-array #1(w286, w288) -> ()  [unwired: 1 out]
                  n102 = local read "ALG MSG  TYPE"() -> (w292:enum16{"void", "byte", "int", "float"})
                  "ALG MSG  PARAM 2" <- w292
                  n103 = property on="ALG MSG  PARAM" class="Str"() -> ("Value"=w293:string)  [unwired: 2 in, 2 out]
                  n104 = property on="ALG MSG  CODE" class="CmbBox"() -> ("Value"=w294:string)  [unwired: 2 in, 2 out]
                  n105 = call "ConvertMsgParameter.vi"("MSG  Type"=w292, "MSG  PARAM"=w293) -> ("Casted Parameter"=w291:i32)
                  n106 = Decimal String To Number(string=w294) -> (number=w295:i32)  [unwired: 2 in, 1 out]
                  n107 = Bundle(w295, "Casted Parameter"=w291, "ALG MSG  TYPE"=w292) -> (w290:T7)  [unwired: 1 in]
                  n108 = in-place-array #1(w290) -> (w285:T6)  [unwired: 1 out]
                }
                n109 = Increment(x=w288) -> (x+1=w287:i32)
                n110 = property on="MSG queue" class="Slide (strict)"("Fill Color"=u32 3381759) -> ()  [unwired: 2 in, 2 out]
                n111 = local write "ALG MSG queue"(w287) -> ()
              }
            }
          }
          event "send voc msg 2": Mouse Down {
            n112 = event-data() -> ()  [unwired: 1 in, 8 out]
            n113 = local read "VOC MSG queue"() -> (w301:i32)
            n114 = Less Or Equal?(x=w301, y=99) -> (x <= y?=w305:bool)
            n115 = case shown="True" w305 {
              tunnel: w301 -> [_ w311]
              tunnel: w297 -> [w306 w309]
              tunnel: [w306 w308] -> w296
              frame False {
                n116 = property on="VOC MSG queue" class="Slide (strict)"("Fill Color"=u32 16711680) -> ()  [unwired: 2 in, 2 out]
              }
              frame True {
                n117 = Increment(x=w311) -> (x+1=w310:i32)
                n118 = local write "VOC MSG queue"(w310) -> ()
                n119 = property on="VOC MSG queue" class="Slide (strict)"("Fill Color"=u32 6618880) -> ()  [unwired: 2 in, 2 out]
                n120 = in-place {
                  n121 = in-place-array #2(w309, w311) -> ()  [unwired: 1 out]
                  n122 = property on="VOC MSG  PARAM" class="Str"() -> ("Value"=w315:string)  [unwired: 2 in, 2 out]
                  n123 = local read "VOC MSG  TYPE"() -> (w314:enum16{"void", "byte", "int", "float"})
                  n124 = property on="VOC MSG  CODE" class="CmbBox"() -> ("Value"=w317:string)  [unwired: 2 in, 2 out]
                  n125 = call "ConvertMsgParameter.vi"("MSG  Type"=w314, "MSG  PARAM"=w315) -> ("Casted Parameter"=w313:i32)
                  n126 = Decimal String To Number(string=w317) -> (number=w318:i32)  [unwired: 2 in, 1 out]
                  n127 = Bundle(w318, "Casted Parameter"=w313, "VOC MSG  TYPE"=w314) -> (w316:T8)  [unwired: 1 in]
                  n128 = in-place-array #2(w316) -> (w308:T6)  [unwired: 1 out]
                }
              }
            }
          }
          event "run": Value Change {
            n129 = event-data() -> ()  [unwired: 1 in, 6 out]
            n130 = property on="run" class="Bool (strict)"() -> ("Value"=w326:bool)  [unwired: 2 in, 2 out]
            n131 = Not(x=w326) -> (.not. x?=w325:bool)
            n132 = property on="stop 2" class="Bool (strict)"("Value"=w325) -> ()  [unwired: 2 in, 2 out]
          }
          event "stop 2": Value Change {
            n133 = event-data() -> ()  [unwired: 1 in, 6 out]
            n134 = property on="stop 2" class="Bool (strict)"() -> ("Value"=w334:bool)  [unwired: 2 in, 2 out]
            n135 = Not(x=w334) -> (.not. x?=w333:bool)
            n136 = property on="run" class="Bool (strict)"("Value"=w333) -> ()  [unwired: 2 in, 2 out]
          }
          event User Event; "Tests List": Value Change {
            n137 = event-data() -> ()  [unwired: 1 in, 3 out]
            n138 = List Folder(path=w343, pattern="*.test") -> (path out=w344:path, filenames=w342:string[])  [unwired: 2 in, 2 out]
            n139 = property on="Tests List" class="LstBox (strict)"("Item Names"=w342) -> ()  [unwired: 2 in, 2 out]
            n140 = Array Size(array=w342) -> (size(s)=w347:i32)
            n141 = Not Equal To 0?(x=w347) -> (x != 0?=w346:bool)
            n142 = case shown="False" w346 {
              tunnel: w342 -> [_ w361]
              tunnel: w344 -> [_ w359]
              tunnel: w339 -> [w348 w350]
              tunnel: [w348 w349] -> w338
              frame False {
              }
              frame True {
                n143 = property on="Tests List" class="LstBox (strict)"() -> ("Value"=w351:i32)  [unwired: 2 in, 2 out]
                n144 = Index Array(array=w361, index=w351) -> (element=w360:string)
                n145 = Build Path(base path=w359, name or relative path=w360) -> (appended path=w358:path)
                n146 = call <vilib>:"Open_Create_Replace File.vi"("file path"=w358) -> ("error out"=w356:errorcluster, "file size (bytes)"=w355:i32, "refnum"=w357:refnum<file>)  [unwired: 7 in, 1 out]
                n147 = Read from Binary File(8:w356, 10:w355, 11:w357) -> (0:w353:errorcluster, 2:w352:string, 3:w354:refnum<file>)  [unwired: 3 in, 1 out]
                n148 = call "FindScriptPorts.vi"("Input FOR VOC"=w350, "Test"=w352) -> ("Result Input FOR VOC"=w349:u8[])
                n149 = Close File(refnum=w354, error in=w353) -> ()  [unwired: 2 out]
                n150 = property on="TEST" class="Str"(error in=w353, "Value"=w352) -> ()  [unwired: 1 in, 2 out]
              }
            }
          }
          event "Set new value\n(ALG ports)": Mouse Down {
            n151 = event-data() -> ()  [unwired: 1 in, 8 out]
            n152 = property on="New value\n(ALG ports)" class="DigNum (strict)"() -> ("Value"=w369:u8)  [unwired: 2 in, 2 out]
            n153 = property on="ALG Input Ports" class="MCListbox (strict)"() -> ("Value"=w370:i32)  [unwired: 2 in, 2 out]
            n154 = control-ref of="ALG Input Ports"() -> (w372:refnum<vi>)
            n155 = call "GUIUpdater.vi"("value"=w369, "Color"=u32 13260, "line"=w370, "MCListbox Refnum"=w372) -> ()
            n156 = in-place {
              in-place-border: w369 -> [w373]
              n157 = in-place-array #3(w365, w370) -> ()  [unwired: 1 out]
              n158 = in-place-array #3(w373) -> (w364:u8[])  [unwired: 1 out]
            }
          }
          event "Set new value (VOC ports)": Mouse Down {
            n159 = event-data() -> ()  [unwired: 1 in, 8 out]
            n160 = property on="VOC Input Ports" class="MCListbox (strict)"() -> ("Value"=w381:i32)  [unwired: 2 in, 2 out]
            n161 = property on="New value (VOC ports)" class="DigNum (strict)"() -> ("Value"=w382:u8)  [unwired: 2 in, 2 out]
            n162 = control-ref of="VOC Input Ports"() -> (w384:refnum<vi>)
            n163 = call "GUIUpdater.vi"("value"=w382, "Color"=u32 39219, "line"=w381, "MCListbox Refnum"=w384) -> ()
            n164 = in-place {
              in-place-border: w382 -> [w385]
              n165 = in-place-array #4(w378, w381) -> ()  [unwired: 1 out]
              n166 = in-place-array #4(w385) -> (w377:u8[])  [unwired: 1 out]
            }
          }
          event "VOC Input Ports": Value Change {
            n167 = event-data() -> ("NewVal"=w393:i32)  [unwired: 1 in, 5 out]
            n168 = Index Array(array=w391, index=w393) -> (element=w392:bool)
            n169 = case shown="True" w392 {
              frame False {
                n170 = property on="Set new value (VOC ports)" class="Bool (strict)"("DisabledEnum"=T2."Disabled and Grayed Out" ("Disabled")) -> ()  [unwired: 2 in, 2 out]
              }
              frame True {
                n171 = property on="Set new value (VOC ports)" class="Bool (strict)"("DisabledEnum"=T2."Enabled" ("Disabled")) -> ()  [unwired: 2 in, 2 out]
              }
            }
            n172 = local write "Controlable (VOC ports)"(w392) -> ()
          }
          event "ALG Input Ports": Value Change {
            n173 = event-data() -> ("NewVal"=w403:i32)  [unwired: 1 in, 5 out]
            n174 = Index Array(array=w401, index=w403) -> (element=w402:bool)
            n175 = local write "Controlable\n(ALG ports)"(w402) -> ()
            n176 = case shown="False" w402 {
              frame False {
                n177 = property on="Set new value\n(ALG ports)" class="Bool (strict)"("DisabledEnum"=T2."Disabled and Grayed Out" ("Disabled")) -> ()  [unwired: 2 in, 2 out]
              }
              frame True {
                n178 = property on="Set new value\n(ALG ports)" class="Bool (strict)"("DisabledEnum"=T2."Enabled" ("Disabled")) -> ()  [unwired: 2 in, 2 out]
              }
            }
          }
          event "Controlable\n(ALG ports)": Value Change {
            n179 = event-data() -> ("NewVal"=w413:bool)  [unwired: 1 in, 5 out]
            n180 = Not(x=w413) -> (.not. x?=w416:bool)
            n181 = Boolean To (0,1)(Boolean=w416) -> (0, 1=w419:i16)
            n182 = Multiply(x=w419, y=i16 2) -> (x*y=w417:i16)
            n183 = property on="ALG Input Ports" class="MCListbox (strict)"() -> ("Value"=w414:i32)  [unwired: 2 in, 2 out]
            n184 = in-place {
              in-place-border: w413 -> [w421]
              n185 = in-place-array #5(w411, w414) -> ()  [unwired: 1 out]
              n186 = in-place-array #5(w421) -> (w412:bool[])  [unwired: 1 out]
            }
            n187 = property on="ALG Input Ports" class="MCListbox (strict)"() -> ("ItemNames"=w415:string[][])  [unwired: 2 in, 2 out]
            n188 = property on="Set new value\n(ALG ports)" class="Bool (strict)"("Disabled"=w417) -> ()  [unwired: 2 in, 2 out]
            n189 = case shown="False" w413 {
              tunnel: w414 -> [w423 w428]
              tunnel: w415 -> [w422 w429]
              tunnel: [w424 w427] -> w420
              frame False {
                n190 = in-place {
                  n191 = in-place-array #6(w422, w423, 1 ("disabled index (col)")) -> ()  [unwired: 1 out]
                  n192 = in-place-array #6("НЕУПР") -> (w424:string[][])  [unwired: 2 out]
                }
              }
              frame True {
                n193 = in-place {
                  n194 = in-place-array #7(w429, w428, 1 ("disabled index (col)")) -> ()  [unwired: 1 out]
                  n195 = in-place-array #7("УПР") -> (w427:string[][])  [unwired: 2 out]
                }
              }
            }
            n196 = property on="ALG Input Ports" class="MCListbox (strict)"("Item Names"=w420) -> ()  [unwired: 2 in, 2 out]
          }
          event "Controlable (VOC ports)": Value Change {
            n197 = event-data() -> ("NewVal"=w439:bool)  [unwired: 1 in, 5 out]
            n198 = Not(x=w439) -> (.not. x?=w442:bool)
            n199 = Boolean To (0,1)(Boolean=w442) -> (0, 1=w445:i16)
            n200 = property on="VOC Input Ports" class="MCListbox (strict)"() -> ("Value"=w438:i32)  [unwired: 2 in, 2 out]
            n201 = in-place {
              in-place-border: w439 -> [w447]
              n202 = in-place-array #8(w440, w438) -> ()  [unwired: 1 out]
              n203 = in-place-array #8(w447) -> (w437:bool[])  [unwired: 1 out]
            }
            n204 = Multiply(x=w445, y=i16 2) -> (x*y=w443:i16)
            n205 = property on="VOC Input Ports" class="MCListbox (strict)"() -> ("ItemNames"=w441:string[][])  [unwired: 2 in, 2 out]
            n206 = property on="Set new value (VOC ports)" class="Bool (strict)"("Disabled"=w443) -> ()  [unwired: 2 in, 2 out]
            n207 = case shown="True" w439 {
              tunnel: w438 -> [w450 w455]
              tunnel: w441 -> [w449 w456]
              tunnel: [w448 w453] -> w446
              frame False {
                n208 = in-place {
                  n209 = in-place-array #9(w449, w450, 1 ("disabled index (col)")) -> ()  [unwired: 1 out]
                  n210 = in-place-array #9("НЕУПР") -> (w448:string[][])  [unwired: 2 out]
                }
              }
              frame True {
                n211 = in-place {
                  n212 = in-place-array #10(w456, w455, 1 ("disabled index (col)")) -> ()  [unwired: 1 out]
                  n213 = in-place-array #10("УПР") -> (w453:string[][])  [unwired: 2 out]
                }
              }
            }
            n214 = property on="VOC Input Ports" class="MCListbox (strict)"("Item Names"=w446) -> ()  [unwired: 2 in, 2 out]
          }
          event "Save changes in current test": Mouse Down {
            w471 = 0 ("pos offset (0)")
            n215 = event-data() -> ()  [unwired: 1 in, 8 out]
            n216 = property on="Tests List" class="LstBox (strict)"() -> ("Value"=w473:i32)  [unwired: 2 in, 2 out]
            n217 = property on="Tests List" class="LstBox (strict)"() -> ("Item Names"=w474:string[])  [unwired: 2 in, 2 out]
            n218 = Index Array(array=w474, index=w473) -> (element=w479:string)
            n219 = Build Path(base path=w475, name or relative path=w479) -> (appended path=w478:path)
            n220 = property on="TEST" class="Str"() -> ("Value"=w468:string)  [unwired: 2 in, 2 out]
            n221 = call <vilib>:"Open_Create_Replace File.vi"("function (open:0)"=T3."open", "file path"=w478) -> ("error out"=w469:errorcluster, "refnum"=w470:refnum<file>)  [unwired: 6 in, 2 out]
            n222 = call "FindScriptPorts.vi"("Input FOR VOC"=w462, "Test"=w468) -> ("Result Input FOR VOC"=w461:u8[])
            n223 = Set File Position(offset (in bytes) (0)=w471, refnum=w470, from (0:start)=w471, error in=w469) -> (refnum out=w467:refnum<file>, error out=w466:errorcluster)
            n224 = Write to Binary File(file (use dialog)=w467, data=w468, error in=w466, 5:FALSE ("prepend array or string size? (T)")) -> (refnum out=w477:refnum<file>, error out=w476:errorcluster)  [unwired: 2 in, 1 out]
            n225 = Close File(refnum=w477, error in=w476) -> ()  [unwired: 2 out]
          }
          event "Save as new test": Mouse Down {
            n226 = event-data() -> ()  [unwired: 1 in, 8 out]
            n227 = call "Save new test"() -> ("Test name"=w490:string, "OK"=w489:bool)  [unwired: 17 in, 1 out]
            n228 = property on="TEST" class="Str"() -> ("Value"=w487:string)  [unwired: 2 in, 2 out]
            n229 = case shown="True" w489 {
              tunnel: w488 -> [_ w497]
              tunnel: w490 -> [_ w504]
              tunnel: w487 -> [_ w495]
              tunnel: w484 -> [w491 w493]
              tunnel: [w491 w492] -> w483
              frame False {
              }
              frame True {
                n230 = Concatenate Strings(w504, ".test" ("string")) -> (w498:string)
                n231 = Build Path(base path=w497, name or relative path=w498) -> (appended path=w499:path)
                n232 = call "FindScriptPorts.vi"("Input FOR VOC"=w493, "Test"=w495) -> ("Result Input FOR VOC"=w492:u8[])
                n233 = call <vilib>:"Open_Create_Replace File.vi"("function (open:0)"=T3."open or create", "file path"=w499) -> ("error out"=w503:errorcluster, "refnum"=w500:refnum<file>)  [unwired: 6 in, 2 out]
                n234 = Write to Binary File(file (use dialog)=w500, data=w495, error in=w503, 5:FALSE ("prepend array or string size? (T)")) -> (refnum out=w501:refnum<file>, error out=w502:errorcluster)  [unwired: 2 in, 1 out]
                n235 = Close File(refnum=w501, error in=w502) -> ()  [unwired: 2 out]
              }
            }
          }
        }
        n236 = property on="run" class="Bool (strict)"() -> ("Value"=w257:bool)  [unwired: 2 in, 2 out]
        n237 = case shown="True" w257 {
          tunnel: w261 -> [_ w561]
          tunnel: w260 -> [_ w560]
          tunnel: w259 -> [_ w559]
          tunnel: w258 -> [_ w558]
          tunnel: w256 -> [w517 w553]
          tunnel: [w517 w552] -> w255
          tunnel: w254 -> [_ w557]
          tunnel: w253 -> [_ w556]
          tunnel: w252 -> [_ w555]
          tunnel: w249 -> [_ w554]
          tunnel: w251 -> [w516 w551]
          tunnel: [w516 w550] -> w250
          tunnel: w245 -> [_ w549]
          tunnel: w246 -> [_ w548]
          tunnel: w243 -> [w515 w547]
          tunnel: [w515 w546] -> w242
          tunnel: w241 -> [w514 w545]
          tunnel: [w514 w544] -> w240
          tunnel: w239 -> [w506 w543]
          tunnel: [w506 w542] -> w238
          tunnel: w237 -> [w513 w541]
          tunnel: [w513 w540] -> w236
          tunnel: w235 -> [w512 w539]
          tunnel: [w512 w538] -> w234
          tunnel: w233 -> [w511 w537]
          tunnel: [w511 w536] -> w218
          tunnel: w232 -> [w510 w535]
          tunnel: [w510 w532] -> w219
          tunnel: w221 -> [w509 w531]
          tunnel: [w509 w528] -> w228
          tunnel: w220 -> [w508 w527]
          tunnel: [w508 w524] -> w229
          tunnel: w230 -> [w507 w523]
          tunnel: [w507 w522] -> w231
          tunnel: w227 -> [_ w521]
          tunnel: w226 -> [_ w520]
          tunnel: w225 -> [_ w519]
          tunnel: w224 -> [_ w518]
          frame False {
          }
          frame True {
            # "Output varables bytes"
            # "Output varables ports"
            # "AY Input varables bytes"
            # "AY Input varables ports"
            n238 = flat-sequence {
              tunnel: w557 -> [w608]
              tunnel: w556 -> [w605]
              tunnel: w555 -> [w607]
              tunnel: w554 -> [w606]
              tunnel: w549 -> [w600]
              tunnel: w548 -> [w599]
              tunnel: w547 -> [w597]
              tunnel: [w577] -> w546
              tunnel: w545 -> [w595]
              tunnel: [w585] -> w544
              tunnel: w543 -> [w593]
              tunnel: [w591] -> w542
              tunnel: w541 -> [w592]
              tunnel: [w590] -> w540
              tunnel: w539 -> [w589]
              tunnel: [w588] -> w538
              tunnel: w537 -> [w567]
              tunnel: [w563] -> w536
              tunnel: w535 -> [w569]
              tunnel: [w565] -> w534
              tunnel: w531 -> [w566]
              tunnel: [w562] -> w530
              tunnel: w527 -> [w568]
              tunnel: [w564] -> w526
              tunnel: w523 -> [w587]
              tunnel: [w586] -> w522
              tunnel: w521 -> [w584]
              tunnel: w520 -> [w583]
              tunnel: w519 -> [w576]
              tunnel: w518 -> [w575]
              tunnel: w553 -> [w646]
              tunnel: [w645] -> w552
              tunnel: w551 -> [w642]
              tunnel: [w643] -> w550
              tunnel: w534 -> [w637]
              tunnel: [w637] -> w533
              tunnel: w530 -> [w636]
              tunnel: [w636] -> w529
              tunnel: w526 -> [w635]
              tunnel: [w635] -> w525
              tunnel: w561 -> [w651]
              tunnel: w560 -> [w650]
              tunnel: w559 -> [w649]
              tunnel: w558 -> [w648]
              tunnel: w533 -> [w661]
              tunnel: [w661] -> w532
              tunnel: w529 -> [w655]
              tunnel: [w655] -> w528
              tunnel: w525 -> [w660]
              tunnel: [w660] -> w524
              frame #0 {
                # "OLD Input for ALG"
                # "Input for ALG"
                # "old Input ports FOR VOC"
                n239 = for {
                  N: 1 -> [_]
                  shift-right: [w631] -> w596
                  shift-left: w597 -> [w632]
                  shift-right: [w630] -> w594
                  shift-left: w595 -> [w625]
                  shift-right: [w628] -> w590
                  shift-left: w592 -> [w629]
                  shift-right: [w626] -> w588
                  shift-left: w589 -> [w627]
                  shift-right: [w622] -> w565
                  shift-left: w569 -> [w624]
                  shift-right: [w620] -> w564
                  shift-left: w568 -> [w623]
                  shift-right: [w618] -> w563
                  shift-left: w567 -> [w621]
                  shift-right: [w617] -> w562
                  shift-left: w566 -> [w619]
                  n240 = call "VOC.vi"("input VOC ports"=w632, "voc states array"=w627, "output VOC ports"=w625, "Input VOC msg Array"=w624, "output VOC msg array"=w623) -> ("Filled voc states array"=w626:cluster{u32, u8}[], "Modified input VOC ports"=w634:u8[], "Modified output VOC ports"=w633:u8[], "Clear Input VOC msg Array"=w622:T6, "output VOC array"=w620:T6)  [unwired: 6 in]
                  n241 = call "CA.vi"("init input ports"=w633, "Alg states"=w629, "output"=w634, "input ALG msg array"=w621, "Output ALG msg array"=w619, "VOC output msg CASHE"=w620) -> ("Output Alg states"=w628:cluster{u32, u8}[], "input ports"=w630:u8[], "modified output ports"=w631:u8[], "Clear input msg Array"=w618:T6, "ALG output array"=w617:T6)  [unwired: 5 in]
                }
                "Result Input FOR VOC" <- w596
                "Array" <- w594
                n242 = call "PSConverter.vi"("Current States 2"=w593, "PROC"=w608, "STATES"=w605, "Input claster"=w590) -> ("Current States"=w591:string[][])
                n243 = property on="Alg States" class="Tbl (strict)"("Value"=w591) -> ()  [unwired: 2 in, 2 out]
                n244 = call "PSConverter.vi"("Current States 2"=w587, "PROC"=w607, "STATES"=w606, "Input claster"=w588) -> ("Current States"=w586:string[][])
                n245 = call "PortsArrayHandler.vi"("Input"=w596, "Init Input"=w597, "INPUT PORT states"=w599) -> ("Rezult Input Ports"=w577:u8[])  [unwired: 1 in]
                n246 = call "PortsArrayHandler.vi"("Input"=w594, "Init Input"=w595, "INPUT PORT states"=w600) -> ("Rezult Input Ports"=w585:u8[])  [unwired: 1 in]
                n247 = local write "VOC States"(w586) -> ()
                n248 = call "FormVarValuesArray.vi"("varables bytes"=w583, "varables ports"=w584, "Ports"=w585) -> ("Values Array"=w580:string[])  [unwired: 1 in]
                n249 = control-ref of="VOC Input Ports"() -> (w603:refnum<vi>)
                n250 = for {
                  tunnel: w603 -> [w611]
                  tunnel: u32 3394560 -> [w610]
                  tunnel: w577 -> [w609] mode=indexing
                  i -> [w612]
                  n251 = call "GUIUpdater.vi"("value"=w609, "Color"=w610, "line"=w612, "MCListbox Refnum"=w611) -> ()
                }
                n252 = local read "AY Input varables names"() -> (w581:string[])
                n253 = local read "AY Input varables type"() -> (w582:string[])
                n254 = call "FormVarValuesArray.vi"("varables bytes"=w575, "varables ports"=w576, "Ports"=w577) -> ("Values Array"=w572:string[])  [unwired: 1 in]
                n255 = local read "Output varables type"() -> (w571:string[])
                n256 = local read "Output varables names"() -> (w570:string[])
                n257 = control-ref of="ALG Input Ports"() -> (w604:refnum<vi>)
                n258 = for {
                  tunnel: w604 -> [w615]
                  tunnel: u32 13260 -> [w614]
                  tunnel: w585 -> [w613] mode=indexing
                  i -> [w616]
                  n259 = call "GUIUpdater.vi"("value"=w613, "Color"=w614, "line"=w616, "MCListbox Refnum"=w615) -> ()
                }
                n260 = Build Array(w582, w581, w580) -> (w579:string[][])
                n261 = Transpose 2D Array(2D array=w579) -> (transposed array=w578:string[][])
                n262 = Build Array(w571, w570, w572) -> (w574:string[][])
                n263 = local write "AY INPUT Variables"(w578) -> ()
                n264 = Transpose 2D Array(2D array=w574) -> (transposed array=w573:string[][])
                n265 = local write "AY OUTPUT Variables"(w573) -> ()
              }
              frame #1 {
                n266 = local read "Curr step VOC MSG counter"() -> (w647:i32)
                n267 = control-ref of="VOC Last Interation MSG"() -> (w640:refnum<vi>)
                n268 = control-ref of="Output VOC Msg LOG"() -> (w641:refnum<vi>)
                n269 = local read "Curr step ALG msg counter"() -> (w644:i32)
                n270 = control-ref of="Output Alg Msg LOG"() -> (w639:refnum<vi>)
                n271 = control-ref of="ALG Last Interation MSG"() -> (w638:refnum<vi>)
                n272 = call "MsgParser.vi"("LAST MSGS"=w640, "MSG LOG"=w641, "MSG Counter"=w646, "current msg num"=w647) -> ("Result Counter"=w645:i32)  [unwired: 1 in]
                n273 = call "MsgParser.vi"("LAST MSGS"=w638, "MSG LOG"=w639, "MSG Counter"=w642, "current msg num"=w644) -> ("Result Counter"=w643:i32)  [unwired: 1 in]
              }
              frame #2 {
                n274 = call "LastStepMsgParser.vi"("Out MSG Names"=w651, "Out MSG Codes"=w650, "Msg Array"=w660) -> ("Output Alg Msg"=w659:string[][], "current msg num"=→"Curr step VOC MSG counter":i32)  [unwired: 5 in, 1 out]
                n275 = property on="VOC Last Interation MSG" class="MCListbox (strict)"("Item Names"=w659) -> ()  [unwired: 2 in, 2 out]
                n276 = call "LastStepMsgParser.vi"("Out MSG Names"=w648, "Out MSG Codes"=w649, "Msg Array"=w655) -> ("Output Alg Msg"=w657:string[][], "current msg num"=→"Curr step ALG msg counter":i32)  [unwired: 5 in, 1 out]
                n277 = property on="ALG Last Interation MSG" class="MCListbox (strict)"("Item Names"=w657) -> ()  [unwired: 2 in, 2 out]
                n278 = local read "Mode"() -> (w654:bool)
                n279 = local read "run"() -> (w653:bool)
                n280 = And(x=w654, y=w653) -> (x .and. y?=w652:bool)
                n281 = case shown="False" w652 {
                  frame False {
                    n282 = local write "stop 2"(TRUE ("stop 2")) -> ()
                    n283 = local write "run"(FALSE ("run")) -> ()
                  }
                  frame True {
                    n284 = local write "stop 2"(FALSE ("stop 2")) -> ()
                    n285 = local write "run"(TRUE ("run")) -> ()
                  }
                }
              }
            }
          }
        }
        n286 = call "FillMsgArray.vi"("Input VOC msg Array"=w229) -> ("Clear msg Array"=w216:T6)
        n287 = call "FillMsgArray.vi"("Input VOC msg Array"=w228) -> ("Clear msg Array"=w217:T6)
      }
    }
  }
